vi "ContourFilled.vi"   [LabVIEW 2013, in "Advanced Plotting Toolkit.lvlib"]
uses:
  Advanced Plotting Toolkit.lvlib
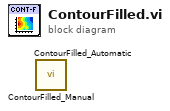
[diagram p0: block diagram]
diagram:
  n1 = call "ContourFilled_Manual.vi"() -> ()  [unwired: 10 in, 2 out]
  n2 = call "ContourFilled_Automatic.vi"() -> ()  [unwired: 10 in, 2 out]
